vi "ReleaseScreen2Normal.vi"(8 "error in (no error)":errorcluster, 11 "Handle in":i64) -> (0 "error out":errorcluster)   [LabVIEW 2020, in "Power Requests.lvlib"]
uses:
  Power Requests.lvlib
  Power Availabilty Requests/Type Defs/Power Request Type.ctl
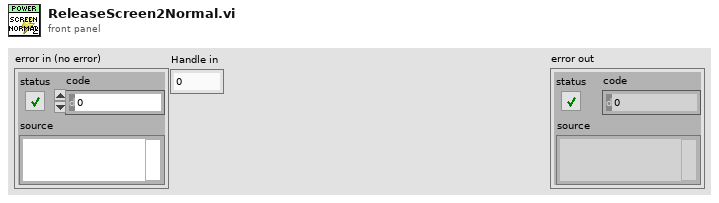
[diagram p1: front panel]
types:
  T1 = typedef "Power Requests.lvlib/Power Request Type.ctl" = enum32{"Power Request Display Required", "Power Request System Required", "Power Request Away Mode Required", "Power Request Execution Required"}
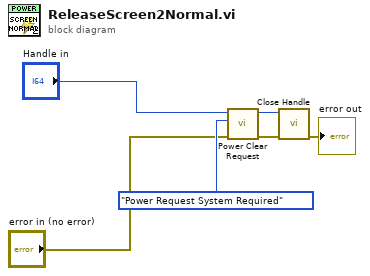
[diagram p0: block diagram]
diagram:
  n1 = call "Power Clear Request.vi"("error in (no error)"="error in (no error)", "Power Request Type"=Power_Request_Type."Power Request System Required", "Handle in"="Handle in") -> ("error out"=w6:errorcluster, "Handle out"=w5:u32)  [unwired: 6 in, 1 out]
  n2 = call "Close Handle.vi"("error in (no error)"=w6, "Handle"=w5) -> ("error out"=→"error out":errorcluster)  [unwired: 8 in, 1 out]
